vi "PID.vi"(7 "继电器":bool=TRUE, 10 "SET":i32[](array[numeric])=[0, 0, 0, 0], 11 "ENC":i32[](array[numeric])=[0, 0, 0, 0, 0, 0, 0]) -> (2 "DIR":bool[](array[boolean]), 3 "PWM":dbl[](array[numeric])=[0.0, 0.0, 0.0, 1.0, 1.0, 1.0, 1.0])   [LabVIEW 2017]
uses:
  <vilib>/addons/control/pid/pid.llb/PID (DBL Array).vi
  <vilib>/addons/control/pid/NI_PID_pid.lvlib
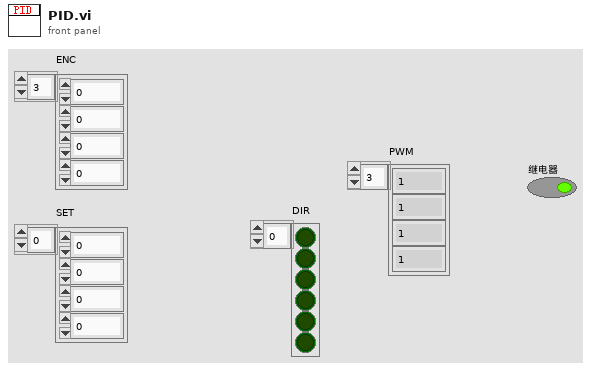
[diagram p1: front panel]
types:
  T1 = cluster{"proportional gain (Kc)":dbl, "integral time (Ti, min)":dbl, "derivative time (Td, min)":dbl}
  T2 = cluster{"proportional gain (Kc)":dbl, "integral time (Ti, min)":dbl, "derivative time (Td, min)":dbl}[]
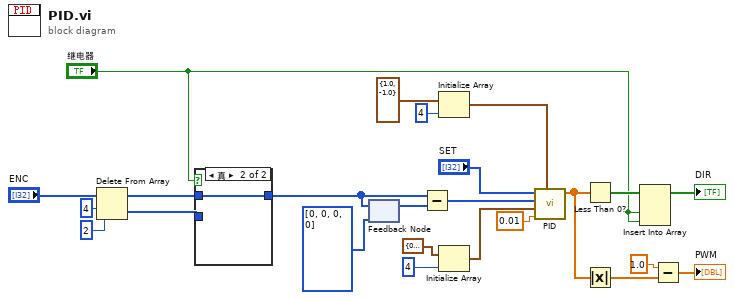
[diagram p0: block diagram]
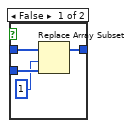
[diagram p2: hidden frame]
diagram:
  n1 = Delete From Array(array="ENC", length=2 ("长度"), index=4 ("索引")) -> (deleted portion=w4:i32[], array with subset deleted=w3:i32[])
  n2 = case shown="真" "继电器" {
    tunnel: w4 -> [w28 _]
    tunnel: w3 -> [w26 w29]
    tunnel: [w25 w29] -> w1
    frame False {
      n3 = Replace Array Subset(array=w26, new element=w28, index=1 ("索引")) -> (w25:i32[])
    }
    frame True {
    }
  }
  n4 = feedback #1(i32[] [0, 0, 0, 0] ("ENC")) -> (w24:i32[])
  n5 = feedback-in #1(w1) -> ()
  n6 = Subtract(x=w1, y=w24) -> (x-y=w12:i32[])
  n7 = Initialize Array(cluster{"output high":dbl, "output low":dbl} {"output high"=1.0, "output low"=-1.0} ("output range"), 4 ("维数大小")) -> (w13:cluster{"output high":dbl, "output low":dbl}[])
  n8 = Initialize Array(T1 {"proportional gain (Kc)"=0.001, "integral time (Ti, min)"=1.8e-05, "derivative time (Td, min)"=0.0} ("PID gains"), 4 ("维数大小")) -> (w16:T2)
  n9 = call-poly <vilib>:"PID.vi"("output range"=w13, "dt (s)"=0.01, "PID gains"=w16, "process variable"=w12, "setpoint"="SET") -> ("output"=w21:dbl[])  [unwired: 5 in, 1 out]
  n10 = Less Than 0?(x=w21) -> (x < 0?=w8:bool[])
  n11 = Absolute Value(x=w21) -> (abs(x)=w20:dbl[])
  n12 = Insert Into Array(array=w8, new element #1="继电器", new element #2="继电器") -> (→"DIR":bool[])  [unwired: 1 in]
  n13 = Subtract(x=1.0, y=w20) -> (x-y=→"PWM":dbl[])
